vi "Initialize-Standard.vi"(5 "Reset? (F: No)":bool=TRUE, 6 "Checksum (Disabled)":bool, 7 "ID Query? (Enabled)":bool=TRUE, 8 "error in (no error)":errorcluster, 9 "Serial Configuration (19200 : 19200 Baud)":u32(ring)=19200 items=["19200"=19200, "57600"=57600, "115200"=115200, "250000"=250000, "500000"=500000, "750000"=750000], 10 "Protocol (2: SCIP 2.0)":u32(ring)=2 items=["Convert to Latest", "SCIP 1.1", "SCIP 2.0"], 11 "VISA resource name":refnum<visa-resource-name>) -> (0 "error out":errorcluster, 3 "VISA resource name out":refnum<visa-resource-name>)   [LabVIEW 2014, in "Hokuyo URG Series.lvlib"]
doc: "Establishes communication with the instrument. It also places the instrument in a default state needed for other instrument driver operations. Therefore, call this VI before calling other instrument driver VIs for this instrument. Generally, you need to call the Initialize VI only once at the beginning of an application."
uses:
  Hokuyo URG Series.lvlib
panel:
  # "(c) 2009 - 2012 National Instruments.  ALL RIGHTS RESERVED."
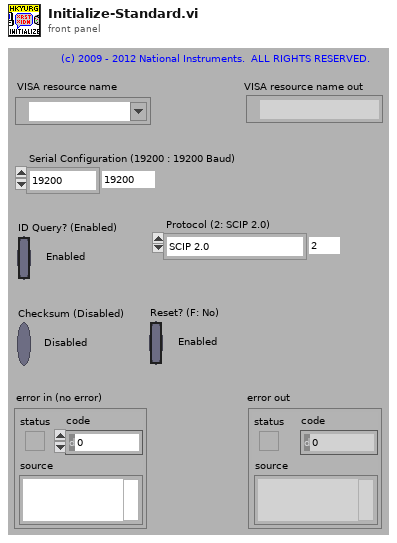
[diagram p1: front panel]
types:
  T1 = cluster{"Sensor Model":string, "Minimum Measurement":string, "Maximum Measurement":string, "Total Steps in Range":string, "First Step in Range":string, "Last Step in Range":string, "Front Step":string, "Standard Motor Speed":string}
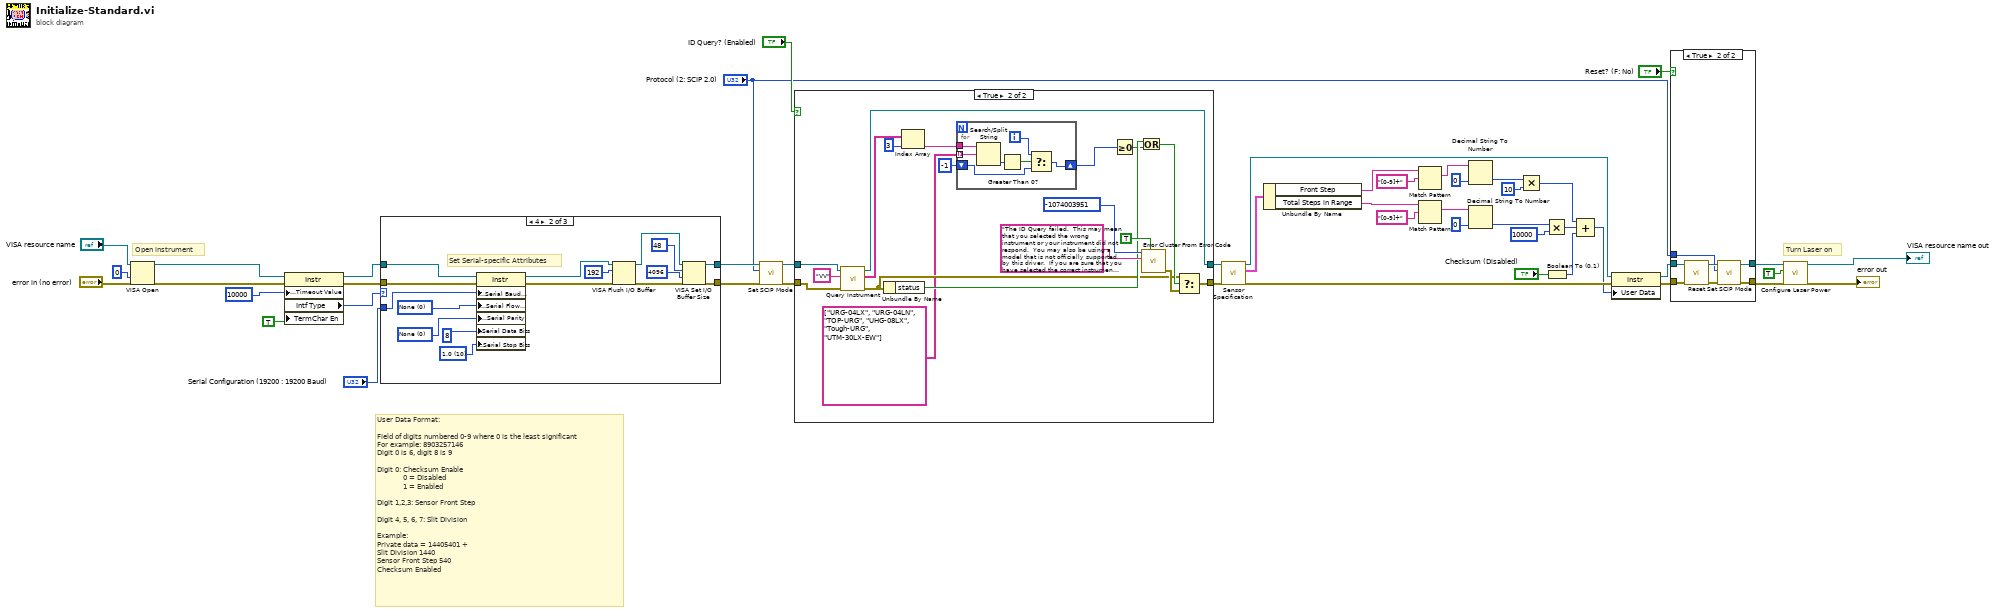
[diagram p0: block diagram]
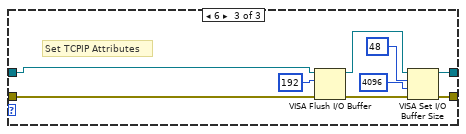
[diagram p3: hidden frame]
diagram:
  # "Open instrument"
  # "User Data Format:\n\nField of digits numbered 0-9 where 0 is the least significant\nFor example: 8903257146\nDigit 0 is 6, digit 8 is 9\n\nDigit 0: Checksum Enable\n             0 = Disabled\n             1 = Enabled\n\nDigit 1,2,3: Sensor Front Step\n\nDigit 4, 5, 6, 7: Slit Division\n\nExample:\nPrivate data = 14405401 +\nSlit Division 1440\nSensor Front Step 540\nChecksum Enabled"
  # "Turn Laser on"
  n1 = VISA Open(access mode=u32 0, error in (no error)="error in (no error)", VISA resource name="VISA resource name") -> (VISA resource name=w11:refnum<visa-resource-name>, error out=w10:errorcluster)  [unwired: 2 out]
  n2 = property class="Instr"(reference=w11, error in=w10, "General Settings:Timeout Value"=u32 10000, "TermChar En"=TRUE) -> (reference out=w46:refnum<visa-resource-name>, error out=w45:errorcluster, "Intf Type"=w1:u16)
  n3 = case shown="4" w1 {
    tunnel: w46 -> [w49 w65 w67]
    tunnel: w45 -> [w48 w64 w66]
    tunnel: "Serial Configuration (19200 : 19200 Baud)" -> [_ w63 _]
    tunnel: [w48 w51 w69] -> w38
    tunnel: [w49 w50 w68] -> w37
    frame 0, Default {
    }
    frame 4 {
      w52 = u16 10 items=["1.0"=10, "1.5"=15, "2.0"=20] ("Serial Settings:Stop Bits")
      w54 = u16 0 items=["None", "Odd", "Even", "Mark", "Space"] ("Serial Settings:Parity")
      w55 = u16 0 items=["None", "XON/XOFF", "RTS/CTS", "XON/XOFF & RTS/CTS", "DTR/DSR", "XON/XOFF & DTR/DSR"] ("Serial Settings:Flow Control")
      # "Set Serial-specific Attributes"
      n4 = property class="Instr"(reference=w65, error in=w64, "Serial Settings:Serial Baud Rate"=w63, "Serial Settings:Serial Flow Control"=w55, "Serial Settings:Serial Parity"=w54, "Serial Settings:Serial Data Bits"=u16 8 ("Serial Settings:Data Bits"), "Serial Settings:Serial Stop Bits"=w52) -> (reference out=w59:refnum<visa-resource-name>, error out=w61:errorcluster)
      n5 = VISA Flush I/O Buffer(VISA resource name=w59, mask (16)=u16 192, error in (no error)=w61) -> (VISA resource name out=w62:refnum<visa-resource-name>, error out=w60:errorcluster)
      n6 = VISA Set I/O Buffer Size(VISA resource name=w62, mask (16)=u16 48, size (4096)=u32 4096 ("size (0)"), error in (no error)=w60) -> (VISA resource name out=w50:refnum<visa-resource-name>, error out=w51:errorcluster)
    }
    frame 6 {
      # "Set TCPIP Attributes"
      n7 = VISA Flush I/O Buffer(VISA resource name=w67, mask (16)=u16 192, error in (no error)=w66) -> (VISA resource name out=w74:refnum<visa-resource-name>, error out=w73:errorcluster)
      n8 = VISA Set I/O Buffer Size(VISA resource name=w74, mask (16)=u16 48, size (4096)=u32 4096 ("size (0)"), error in (no error)=w73) -> (VISA resource name out=w68:refnum<visa-resource-name>, error out=w69:errorcluster)
    }
  }
  n9 = call "Set SCIP Mode.vi"("error in (no error)"=w38, "Protocol (2: SCIP 2.0)"="Protocol (2: SCIP 2.0)", "VISA resource name"=w37) -> ("error out"=w35:errorcluster, "VISA resource name out"=w36:refnum<visa-resource-name>)  [unwired: 7 in]
  n10 = case shown="True" "ID Query? (Enabled)" {
    tunnel: w36 -> [w76 w86]
    tunnel: w35 -> [w75 w85]
    tunnel: [w76 w83] -> w32
    tunnel: [w75 w82] -> w30
    frame False {
    }
    frame True {
      n11 = call "Query Instrument.vi"("error in"=w85, "Command"="VV", "VISA Resource Name"=w86) -> ("error out"=w84:errorcluster, "Response Strings"=w87:string[], "VISA Resource Name Out"=w83:refnum<visa-resource-name>)  [unwired: 6 in]
      n12 = Unbundle By Name(w84) -> ("status"=w91:bool)
      n13 = Index Array(array=w87, index=3) -> (element=w79:string)
      n14 = for {
        tunnel: string[] ["URG-04LX", "URG-04LN", "TOP-URG", "UHG-08LX", "Tough-URG", "UTM-30LX-EW"] -> [w102] mode=indexing
        tunnel: w79 -> [w101]
        shift-right: [w98] -> w78
        shift-left: -1 ("offset of match") -> [w97]
        i -> [w96]
        n15 = Search/Split String(string=w101, search string/char (-)=w102) -> (offset of match=w100:i32)  [unwired: 1 in, 2 out]
        n16 = Greater Than 0?(x=w100) -> (x > 0?=w99:bool)
        n17 = Select(t=w96, s=w99, f=w97) -> (s? t:f=w98:i32)
      }
      n18 = Greater Or Equal To 0?(x=w78) -> (x >= 0?=w90:bool)
      n19 = Or(x=w91, y=w90) -> (x .or. y?=w89:bool)
      n20 = call <vilib>:"Error Cluster From Error Code.vi"("show call chain? (False)"=TRUE, "error message (\"\")"="The ID Query failed.  This may mean that you selected the wrong instrument or your instrument did not respond.  You may also be using a model that is not officially supported by this driver.  If you are sure that you have selected the correct instrument and it is responding, try disabling the ID Query." ("Source (VI Name)"), "error code (0)"=-1074003951 ("Code")) -> ("error out"=w95:errorcluster)  [unwired: 1 in, 5 out]
      n21 = Select(t=w84, s=w89, f=w95) -> (s? t:f=w82:errorcluster)
    }
  }
  n22 = call "Sensor Specification.vi"("error in (no error)"=w30, "VISA resource name"=w32) -> ("error out"=w31:errorcluster, "Instrument Specifications"=w29:T1, "VISA resource name out"=w33:refnum<visa-resource-name>)  [unwired: 7 in]
  n23 = Unbundle By Name(w29) -> ("Front Step"=w18:string, "Total Steps in Range"=w14:string)
  n24 = Match Pattern(string=w18, regular expression="[0-9]+") -> (match substring=w16:string)  [unwired: 1 in, 3 out]
  n25 = Match Pattern(string=w14, regular expression="[0-9]+") -> (match substring=w13:string)  [unwired: 1 in, 3 out]
  n26 = Decimal String To Number(string=w16, default (0L)=u32 0 ("default (0 I32)")) -> (number=w26:u32)  [unwired: 1 in, 1 out]
  n27 = Decimal String To Number(string=w13, default (0L)=u32 0 ("default (0 I32)")) -> (number=w25:u32)  [unwired: 1 in, 1 out]
  n28 = Multiply(x=w26, y=u32 10) -> (x*y=w20:u32)
  n29 = Multiply(x=w25, y=u32 10000) -> (x*y=w21:u32)
  n30 = Boolean To (0,1)(Boolean="Checksum (Disabled)") -> (0, 1=w22:i16)
  n31 = Compound Arithmetic op=ADD(w20, w21, w22) -> (w19:u32)
  n32 = property class="Instr"(reference=w33, error in=w31, "User Data"=w19) -> (reference out=w7:refnum<visa-resource-name>, error out=w5:errorcluster)
  n33 = case shown="True" "Reset? (F: No)" {
    tunnel: w7 -> [w104 w110]
    tunnel: w5 -> [w103 w111]
    tunnel: [w103 w106] -> w4
    tunnel: [w104 w108] -> w6
    tunnel: "Protocol (2: SCIP 2.0)" -> [_ w105]
    frame False {
    }
    frame True {
      n34 = call "Reset.vi"("error in (no error)"=w111, "VISA resource name"=w110) -> ("error out"=w107:errorcluster, "VISA resource name out"=w109:refnum<visa-resource-name>)  [unwired: 8 in]
      n35 = call "Set SCIP Mode.vi"("error in (no error)"=w107, "Protocol (2: SCIP 2.0)"=w105, "VISA resource name"=w109) -> ("error out"=w106:errorcluster, "VISA resource name out"=w108:refnum<visa-resource-name>)  [unwired: 7 in]
    }
  }
  n36 = call "Configure Laser Power.vi"("error in (no error)"=w4, "Laser Power"=TRUE ("Laser"), "VISA resource name"=w6) -> ("error out"=→"error out":errorcluster, "VISA resource name out"=→"VISA resource name out":refnum<visa-resource-name>)  [unwired: 7 in]
